vi "Target Generate Square Wave Torque Setpoint.vi"(11 "Torque Square Wave Parameters":T2) -> (0 "Phase Array (0-1)":dbl[](array[numeric]), 3 "Square Wave (Nm)":dbl[](array[numeric]))   [LabVIEW 2018, in "COBRA Torque Setpoint Generators Library.lvlib"]
uses:
  COBRA Torque Setpoint Generators Library.lvlib
  Square Wave Torque Parameters.ctl
  <vilib>/Analysis/1siggen.llb/Ramp Pattern by Samples.vi
  <vilib>/Analysis/NI_AALBase.lvlib
panel:
  out "XY Graph":T1(graph)
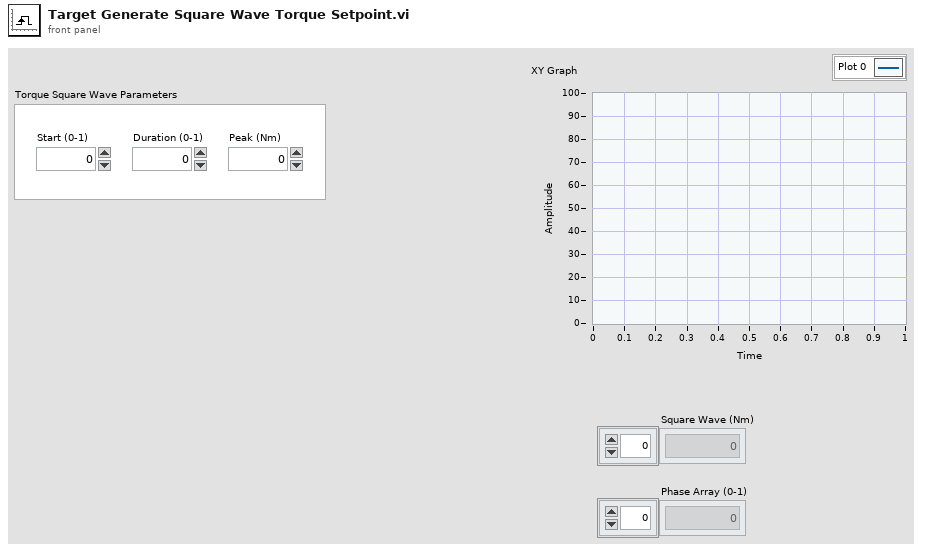
[diagram p1: front panel]
types:
  T1 = cluster{"Ramp Pattern":dbl[], "square wave":dbl[]}
  T2 = typedef "COBRA Torque Setpoint Generators Library.lvlib/Square Wave Torque Parameters.ctl" = cluster{"Start (0-1)":dbl, "Duration (0-1)":dbl, "Peak (Nm)":dbl}
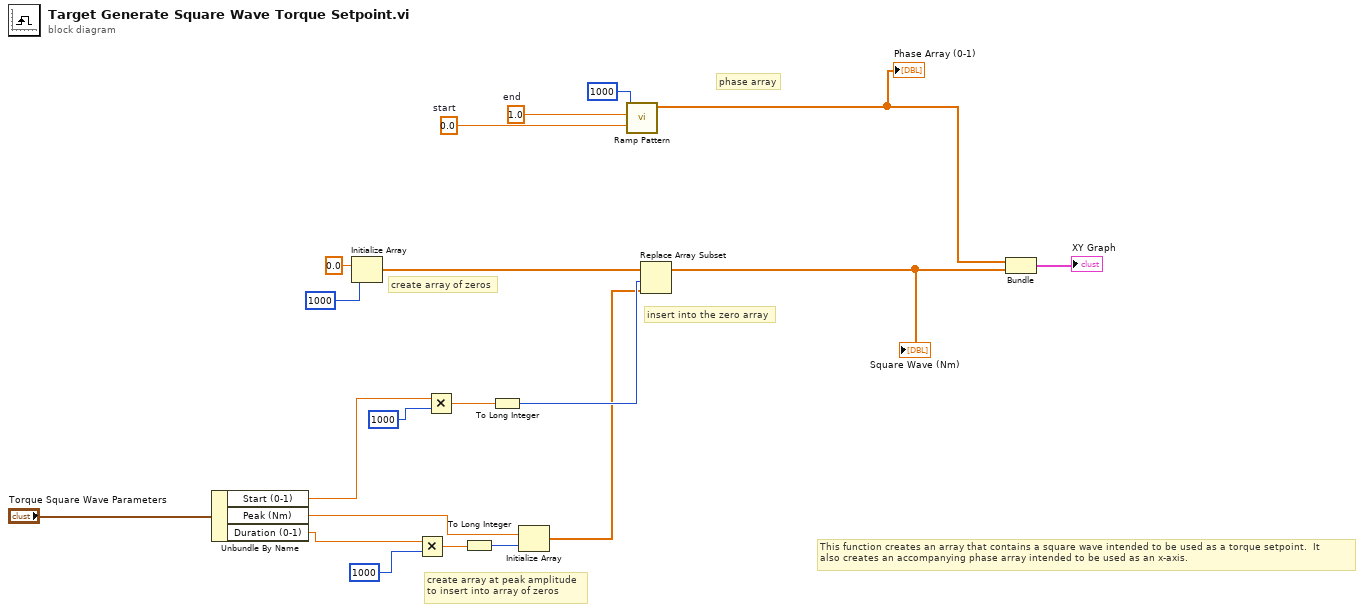
[diagram p0: block diagram]
diagram:
  w18 = 0.0  # start
  w19 = 1.0  # end
  # "phase array"
  # "insert into the zero array"
  # "create array at peak amplitude\nto insert into array of zeros"
  # "create array of zeros"
  # "This function creates an array that contains a square wave intended to be used as a torque setpoint.  It\nalso creates an accompanying phase array intended to be used as an x-axis."
  n1 = Unbundle By Name("Torque Square Wave Parameters") -> ("Start (0-1)"=w7:dbl, "Peak (Nm)"=w4:dbl, "Duration (0-1)"=w3:dbl)
  n2 = Initialize Array "Initialize Array"(0.0 ("element"), 1000 ("dimension size")) -> (w13:dbl[])
  n3 = Multiply(x=w3, y=1000 ("dimension size")) -> (x*y=w11:dbl)
  n4 = Multiply(x=w7, y=1000 ("dimension size")) -> (x*y=w6:dbl)
  n5 = To Long Integer(number=w11) -> (32bit integer=w10:i32)
  n6 = To Long Integer(number=w6) -> (32bit integer=w5:i32)
  n7 = Initialize Array "Initialize Array"(w4, w10) -> (w2:dbl[])
  n8 = call-poly <vilib>:"Ramp Pattern.vi"("start"=w18, "end"=w19, "samples"=1000) -> ("Ramp Pattern"=w1:dbl[])  [unwired: 7 in, 1 out]
  "Phase Array (0-1)" <- w1
  n9 = Replace Array Subset "Replace Array Subset"(array=w13, new element=w2, index=w5) -> (w12:dbl[])
  "Square Wave (Nm)" <- w12
  n10 = Bundle("Ramp Pattern"=w1, w12) -> (→"XY Graph":cluster{"Ramp Pattern":dbl[], dbl[]})  [unwired: 1 in]
